vi "Remote Front Panel Test.vi"() -> ()   [LabVIEW 2009]
uses:
  <vilib>/Platform/TimedLoop/XDataNode/XDataNode.xnode
  <vilib>/Platform/TimedLoop/XDataNode/loadlvalarms.vi
  <vilib>/Platform/TimedLoop/XDataNode/timing_clust.ctl
  <vilib>/Platform/TimedLoop/XDataNode/nitl_modes.ctl
  <vilib>/Platform/TimedLoop/XDataNode/wakeup.ctl
  <vilib>/Platform/TimedLoop/XDataNode/XDNodeRunTimeDep.lvlib
panel:
  out "Create Time":timestamp
  in  "stop":bool
  out "Numeric":i32
  out "Remote Panel Connections":T1(array[cluster])
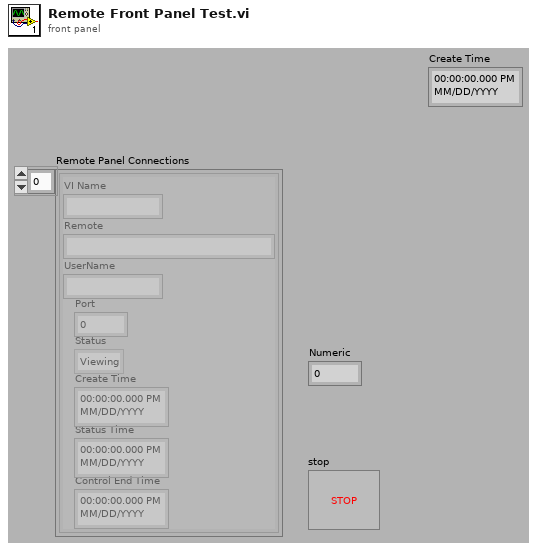
[diagram p1: front panel]
types:
  T1 = cluster{"VI Name":string, "Remote":string, "UserName":string, "Port":i32, "Status":enum32{"Viewing", "Waiting For Control", "Controlling"}, "Create Time":timestamp, "Status Time":timestamp, "Control End Time":timestamp}[]
  T2 = typedef "XDNodeRunTimeDep.lvlib/timing_clust.ctl" = cluster{"Expected End [f-1]":u64, "Actual End [f-1]":u64, "Finished Late? [f-1]":bool, "Expected End [i-1]":u64, "Actual End [i-1]":u64, "Finished Late? [i-1]":bool, "Expected Start [i]":u64, "Actual Start [i]":u64, "Expected Start [f]":u64, "Actual Start [f]":u64, "Source Name":string, "Structure Name":string, "Period":i64, "Deadline":i64, "Offset":i64, "Start":i64, "Priority":i32, "Timeout":i32, "Mode":T3, "Wakeup Reason":T4, "Error":errorcluster, "Source Type":string, "Secondary Source Type":string, "Global End Time":u64, "Global Start Time":u64, "Frame Duration":u64, "Iteration Duration":u64, "Assigned CPU":i32, "I/O Scan Engine Mode":u32}
  T3 = typedef "XDNodeRunTimeDep.lvlib/nitl_modes.ctl" = enum32{"No Change", "Process missed periods, maintain original phase", "Discard missed periods, maintain original phase", "Process missed periods, ignore original phase", "Discard missed periods, ignore original phase"}
  T4 = typedef "XDNodeRunTimeDep.lvlib/wakeup.ctl" = enum32{"Normal", "Aborted", "Asynchronous wakeup", "Timing source error", "Timed loop error", "Timeout"}
  T5 = typedef "LVRemotePanelConnectionsTypeDef.ctl" = cluster{"VI Name":string, "Remote":string, "UserName":string, "Port":i32, "Status":enum32{"Viewing", "Waiting For Control", "Controlling"}, "Create Time":timestamp, "Status Time":timestamp, "Control End Time":timestamp}[]
  T6 = cluster{"VI Name":string, "Remote":string, "UserName":string, "Port":i32, "Status":enum32{"Viewing", "Waiting For Control", "Controlling"}, "Create Time":timestamp, "Status Time":timestamp, "Control End Time":timestamp}
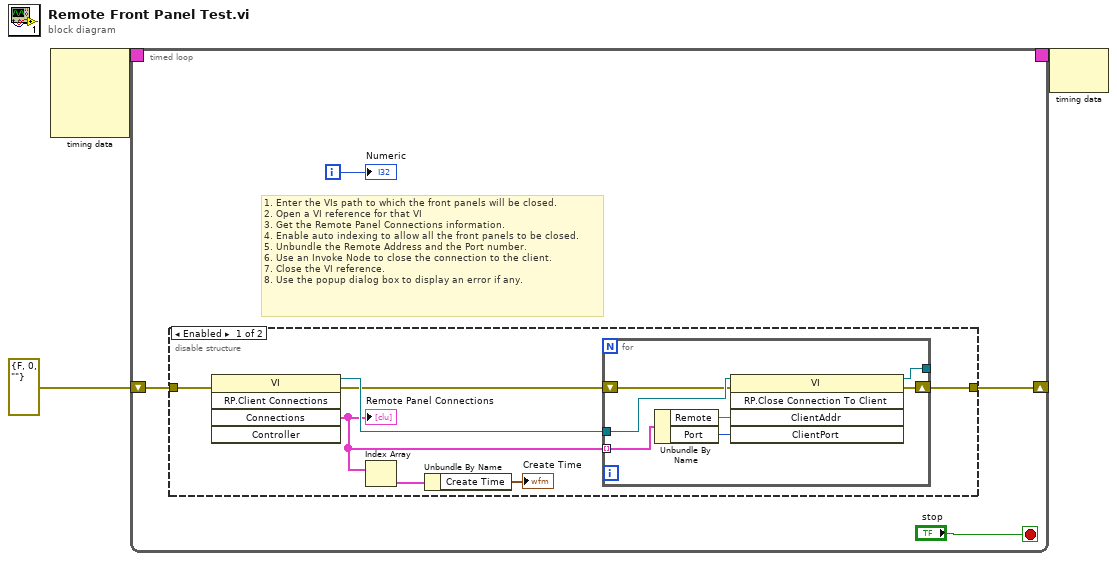
[diagram p0: block diagram]
diagram:
  n1 = node-c288() -> (w3:T2)  [unwired: 4 in]
  n2 = timed-loop {
    timing: w3 -> [_]
    timing-out: [_] -> w2
    shift-right: [w6] -> _
    shift-left: errorcluster {"status"=FALSE, "code"=0, "source"=""} ("error out") -> [w5]
    i -> [w7]
    stop <- "stop" stop-if-true
    # "1. Enter the VIs path to which the front panels will be closed.\n2. Open a VI reference for that VI\n3. Get the Remote Panel Connections information.\n4. Enable auto indexing to allow all the front panels to be closed.\n5. Unbundle the Remote Address and the Port number.\n6. Use an Invoke Node to close the connection to the client.\n7. Close the VI reference.\n8. Use the popup dialog box to display an error if any."
    n3 = disable-structure shown="Enabled" {
      disable-tunnel: [w12 w22] -> w6
      disable-tunnel: w5 -> [w11 w22]
      frame #0 {
        n4 = invoke class="VI" method="RP.Client Connections"(error in=w11) -> (reference out=w14:refnum<vi>, error out=w13:errorcluster, "Connections"=w10:T5)  [unwired: 4 in, 2 out]
        "Remote Panel Connections" <- w10
        n5 = Index Array(array=w10) -> (element=w9:T6)  [unwired: 1 in]
        n6 = Unbundle By Name(w9) -> ("Create Time"=→"Create Time":timestamp)
        n7 = for {
          tunnel: w10 -> [w21] mode=indexing
          shift-right: [w17] -> w12
          shift-left: w13 -> [w19]
          tunnel: w14 -> [w20]
          tunnel: [w18] -> _
          n8 = Unbundle By Name(w21) -> ("Remote"=w15:string, "Port"=w16:i32)
          n9 = invoke class="VI" method="RP.Close Connection To Client"(reference=w20, error in=w19, "ClientAddr"=w15, "ClientPort"=w16) -> (reference out=w18:refnum<vi>, error out=w17:errorcluster)  [unwired: 1 in, 3 out]
        }
      }
      frame #1 {
      }
    }
    "Numeric" <- w7
  }
  n10 = node-c288(w2) -> ()  [unwired: 1 out]
